vi "Initialize Digital Module.vi"(7 "Direction":enum16{"Input", "Output"}(ring), 8 "error in (no error)":errorcluster, 9 "Speed":enum16{"High Speed", "Low Speed"}(ring), 10 "Channels":u8, 11 "Module in":refnum<class "Module.lvclass">) -> (0 "error out":errorcluster, 3 "Module out":refnum<class "Module.lvclass">)   [LabVIEW 2015, in "Module.lvclass"]
uses:
  Module.lvclass
  Module Configuration.ctl
  Module.lvclass/Module.ctl
  VI/Module Loop/Module Loop.lvclass
  <vilib>/Utility/Data Type/NI_Data Type.lvlib
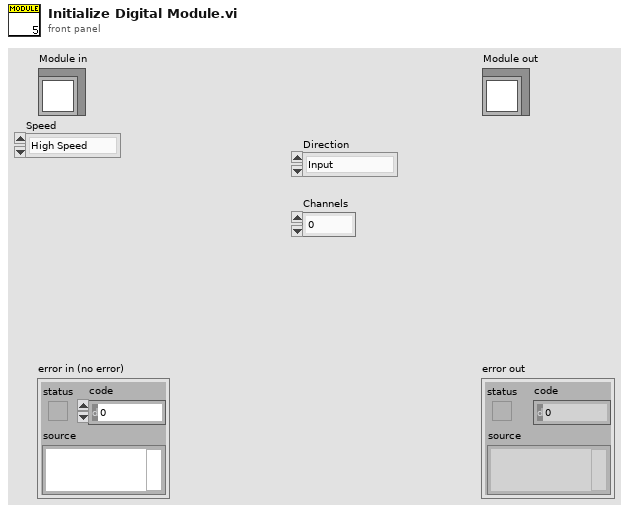
[diagram p1: front panel]
types:
  T1 = typedef "Module Loop.lvclass/Module Configuration.ctl" = cluster{"Type":string, "Direction":string, "Speed":string, "Channels":string, "FXP Type":string}
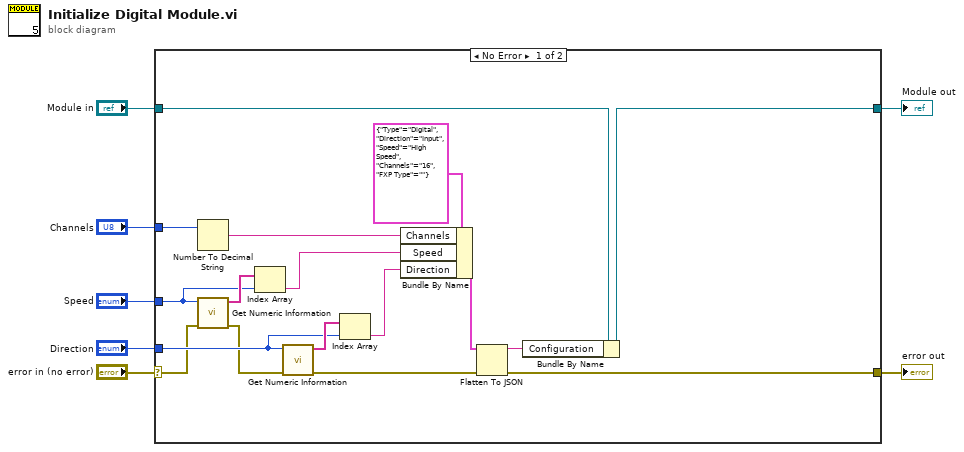
[diagram p0: block diagram]
diagram:
  n1 = case shown="No Error" "error in (no error)" {
    selector: "error in (no error)" -> [w11 w26]
    tunnel: [w21 w26] -> w6
    tunnel: [w17 w25] -> w4
    tunnel: "Module in" -> [w18 w25]
    tunnel: "Direction" -> [w14 _]
    tunnel: "Channels" -> [w23 _]
    tunnel: "Speed" -> [w10 _]
    frame No Error {
      n2 = Number To Decimal String(number=w23) -> (decimal integer string=w22:string)  [unwired: 1 in]
      n3 = call <vilib>:"Get Numeric Information.vi"("error in (no error)"=w11, "Variant"=w10) -> ("error out"=w9:errorcluster, "Enum Names"=w12:string[])  [unwired: 6 in, 2 out]
      n4 = Index Array(array=w12, index=w10) -> (element=w8:string)
      n5 = call <vilib>:"Get Numeric Information.vi"("error in (no error)"=w9, "Variant"=w14) -> ("error out"=w15:errorcluster, "Enum Names"=w16:string[])  [unwired: 6 in, 2 out]
      n6 = Index Array(array=w16, index=w14) -> (element=w13:string)
      n7 = Bundle By Name(cluster=T1 {"Type"="Digital", "Direction"="Input", "Speed"="High Speed", "Channels"="16", "FXP Type"=""} ("Cluster"), "Channels"=w22, "Speed"=w8, "Direction"=w13) -> (w20:T1)
      n8 = Flatten To JSON(anything=w20, error in (no error)=w15) -> (JSON string=w19:string, 11:w21:errorcluster)  [unwired: 1 in]
      n9 = Bundle By Name(cluster=w18, "Configuration"=w19) -> (w17:refnum<class "Module.lvclass">)
    }
    frame Error {
    }
  }
  "error out" <- w6
  "Module out" <- w4
